vi "set_Al_PID_00.vi"(0 "target flow (sccm)":dbl=76.0 format="%.2f", 1 "Run":bool, 2 "Bubbler In":bool, 3 "Active":bool=TRUE) -> ()   [LabVIEW 2011]
uses:
  <vilib>/Analysis/NI_AALPro.lvlib
panel:
  out "prev dR":dbl
  out "dR":dbl
  out "Polynomial Coefficients":dbl[](array[numeric])=[-1.4185856873488687, 0.3207828308209371, 0.13144453708617976]
  out "Best Polynomial Fit":dbl[](array[numeric])=[-1.4185856873488687, -1.6139263817489564, -1.4535753275096295, -0.934721257482187, -0.06084472416107456, 1.168009538292087, 2.7539547788012695, 4.6979090060566655, 6.9965349595828625, 9.65378216839643, 12.656869913925354, 16.032582856357365, 19.766321537116767, 23.839791139200322, 28.29201256813708, 33.090057519195085, 38.231169600301214, 43.741895001434145, 49.604230522561835, 55.817258155180305, 63.621549699110574, 70.69684374251437, 78.07805746158404, 85.78401348130417, 93.89514333055536, 102.37353612475415, 111.1585051750553, 120.33168859799997, 129.86351160527155, 139.71949074374146, 149.9584374415381, 160.56464392932688, 171.50086747103902, 182.82343196442633, 194.50463604214053, 206.47125485701025, 218.94296295023602, 231.70008578092185, 244.74755627283324, 258.3136303817438]
  out "tFit_array":dbl[](array[numeric])=[-2.0, 0.0]
  out "RFit_array":dbl[](array[numeric])=[73.96843433835814, 74.61000000000001]
  out "error array":dbl[](array[numeric])=[-1.3899999999999864, -1.7800000000000011, -1.3500000000000085, -0.6200000000000045, 0.5699999999999932, 1.6099999999999994, 1.1999999999999886, 0.3199999999999932, -0.13000000000000966, -1.3700000000000045, -1.9499999999999886, -1.7399999999999949, -1.1200000000000045, -0.11999999999999034, 1.759999999999991, 2.3500000000000085, 2.1700000000000017, 1.4099999999999966, 0.4299999999999926, -0.6500000000000057, 54.959999999999994, 55.099999999999994, 55.66000000000001, 56.55000000000001, 57.02000000000001, 58.03, 58.129999999999995, 57.11999999999999, 56.599999999999994, 55.47, 54.80000000000001, 54.84, 55.129999999999995, 55.58, 57.16000000000001, 58.11, 58.09, 57.510000000000005, 56.74000000000001, 55.709999999999994]
  out "dt array":dbl[](array[numeric])=[0.0, -1.1669999999867287, -2.3260000000009313, -3.4940000000060536, -4.657999999995809, -5.820999999996275, -6.98499999998603, -8.14999999999418, -9.314000000013039, -10.478999999992084, -11.64000000001397, -12.807000000000698, -13.973999999987427, -15.135999999998603, -16.304000000003725, -17.469000000011874, -18.630999999993946, -19.796000000002095, -20.95999999999185, -22.122999999992317, -23.497999999992317, -24.67499999998836, -25.84299999999348, -27.005999999993946, -28.176000000006752, -29.347000000008848, -30.510999999998603, -31.679000000003725, -32.84700000000885, -34.0109999999986, -35.178000000014435, -36.345999999990454, -37.5109999999986, -38.679000000003725, -39.84700000000885, -41.00800000000163, -42.18299999998999, -43.35099999999511, -44.513000000006286, -45.68900000001304]
  out "Rtarget array":dbl[](array[numeric])=[76.0, 76.0, 76.0, 76.0, 76.0, 76.0, 76.0, 76.0, 76.0, 76.0, 76.0, 76.0, 76.0, 76.0, 76.0, 76.0, 76.0, 76.0, 76.0, 76.0, 20.0, 20.0, 20.0, 20.0, 20.0, 20.0, 20.0, 20.0, 20.0, 20.0, 20.0, 20.0, 20.0, 20.0, 20.0, 20.0, 20.0, 20.0, 20.0, 20.0]
  out "t array":dbl[](array[numeric])=[161845.394, 161844.227, 161843.068, 161841.9, 161840.736, 161839.573, 161838.409, 161837.244, 161836.08, 161834.915, 161833.754, 161832.587, 161831.42, 161830.258, 161829.09, 161827.925, 161826.763, 161825.598, 161824.434, 161823.271, 161821.896, 161820.719, 161819.551, 161818.388, 161817.218, 161816.047, 161814.883, 161813.715, 161812.547, 161811.383, 161810.216, 161809.048, 161807.883, 161806.715, 161805.547, 161804.386, 161803.211, 161802.043, 161800.881, 161799.705]
  out "R array":dbl[](array[numeric])=[74.61000000000001, 74.22, 74.64999999999999, 75.38, 76.57, 77.61, 77.19999999999999, 76.32, 75.86999999999999, 74.63, 74.05000000000001, 74.26, 74.88, 75.88000000000001, 77.75999999999999, 78.35000000000001, 78.17, 77.41, 76.42999999999999, 75.35, 74.96, 75.1, 75.66000000000001, 76.55000000000001, 77.02000000000001, 78.03, 78.13, 77.11999999999999, 76.6, 75.47, 74.80000000000001, 74.84, 75.13, 75.58, 77.16000000000001, 78.11, 78.09, 77.51, 76.74000000000001, 75.71]
  out "tuning":bool
  in  "Tune":bool
  in  "stop":bool
  in  "Ks":dbl
  out "dt(s)":dbl=1.1669999999867287
  out "windup error":dbl
  out "tPrev":dbl=161845.394
  out "target value":dbl=8.607079070006002
  out "error":dbl=-1.3899999999999864
  out "tStart(s)":dbl=161845.394
  out "weight array":dbl[](array[numeric])=[1.0, 0.3112994401423479, 0.09768570948263659, 0.03037911236430853, 0.009485414272106564, 0.0029646390229553033, 0.0009256632966347818, 0.00028873535962988374, 9.01532101455707e-05, 2.8120829299984297e-05, 8.806680295207305e-06, 2.741514645410681e-06, 8.534319742583924e-07, 2.6700458671159456e-07, 8.303530152421186e-08, 2.5900592293904588e-08, 8.103255033572197e-09, 2.5275888811806865e-09, 7.892010589399871e-10, 2.4666252724157755e-10, 6.236605368793774e-11, 1.9221339918994332e-11, 5.977611753902341e-12, 1.8682854076081917e-12, 5.79854027362869e-13, 1.7978764328562998e-13, 5.613594818436806e-14, 1.74576228867237e-14, 5.429116398891195e-15, 1.6951587510987664e-15, 5.277019701540894e-16, 1.6410913665416056e-16, 5.1189358768628024e-17, 1.5919291471855112e-17, 4.95071333304516e-18, 1.5504290109481995e-18, 4.788019052453027e-19, 1.4890178877471836e-19, 4.6585389077974155e-20, 1.437207306183795e-20]
  in  "# of points to watch":i32=60
  in  "tSmooth(s)":dbl=1.0
  out "first":bool
  out "XY Graph":cluster{"Value":dbl[], "Value":dbl[]}[](graph)=[{"Value"=[0.0, -1.1669999999867287, -2.3260000000009313, -3.4940000000060536, -4.657999999995809, -5.820999999996275, -6.98499999998603, -8.14999999999418, -9.314000000013039, -10.478999999992084, -11.64000000001397, -12.807000000000698, -13.973999999987427, -15.135999999998603, -16.304000000003725, -17.469000000011874, -18.630999999993946, -19.796000000002095, -20.95999999999185, -22.122999999992317, -23.497999999992317, -24.67499999998836, -25.84299999999348, -27.005999999993946, -28.176000000006752, -29.347000000008848, -30.510999999998603, -31.679000000003725, -32.84700000000885, -34.0109999999986, -35.178000000014435, -36.345999999990454, -37.5109999999986, -38.679000000003725, -39.84700000000885, -41.00800000000163, -42.18299999998999, -43.35099999999511, -44.513000000006286, -45.68900000001304], "Value"=[74.61000000000001, 74.22, 74.64999999999999, 75.38, 76.57, 77.61, 77.19999999999999, 76.32, 75.86999999999999, 74.63, 74.05000000000001, 74.26, 74.88, 75.88000000000001, 77.75999999999999, 78.35000000000001, 78.17, 77.41, 76.42999999999999, 75.35, 74.96, 75.1, 75.66000000000001, 76.55000000000001, 77.02000000000001, 78.03, 78.13, 77.11999999999999, 76.6, 75.47, 74.80000000000001, 74.84, 75.13, 75.58, 77.16000000000001, 78.11, 78.09, 77.51, 76.74000000000001, 75.71]}, {"Value"=[-2.0, 0.0], "Value"=[73.96843433835814, 74.61000000000001]}, {"Value"=[0.0, -1.1669999999867287, -2.3260000000009313, -3.4940000000060536, -4.657999999995809, -5.820999999996275, -6.98499999998603, -8.14999999999418, -9.314000000013039, -10.478999999992084, -11.64000000001397, -12.807000000000698, -13.973999999987427, -15.135999999998603, -16.304000000003725, -17.469000000011874, -18.630999999993946, -19.796000000002095, -20.95999999999185, -22.122999999992317, -23.497999999992317, -24.67499999998836, -25.84299999999348, -27.005999999993946, -28.176000000006752, -29.347000000008848, -30.510999999998603, -31.679000000003725, -32.84700000000885, -34.0109999999986, -35.178000000014435, -36.345999999990454, -37.5109999999986, -38.679000000003725, -39.84700000000885, -41.00800000000163, -42.18299999998999, -43.35099999999511, -44.513000000006286, -45.68900000001304], "Value"=[76.0, 76.0, 76.0, 76.0, 76.0, 76.0, 76.0, 76.0, 76.0, 76.0, 76.0, 76.0, 76.0, 76.0, 76.0, 76.0, 76.0, 76.0, 76.0, 76.0, 20.0, 20.0, 20.0, 20.0, 20.0, 20.0, 20.0, 20.0, 20.0, 20.0, 20.0, 20.0, 20.0, 20.0, 20.0, 20.0, 20.0, 20.0, 20.0, 20.0]}]
  out "current value":dbl=8.607079070006002
  in  "Period (s)":dbl=0.5
  out "dValue":dbl=2.1714937580001004
  out "derivative":dbl=0.3207828308209371
  out "integral":dbl=21701.037580001004
  in  "Kd":dbl
  in  "Ki":dbl=0.0001
  in  "Kp":dbl=0.001
  out "actual flow (sccm)":dbl=74.61000000000001 format="%.2f"
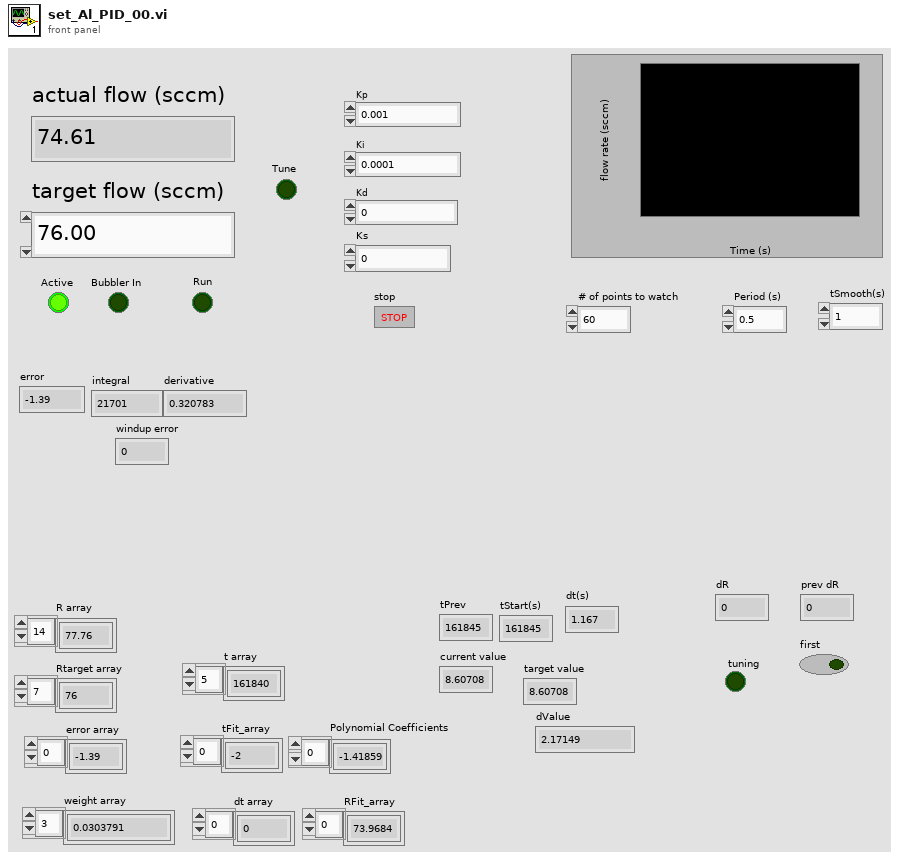
[diagram p1: front panel]
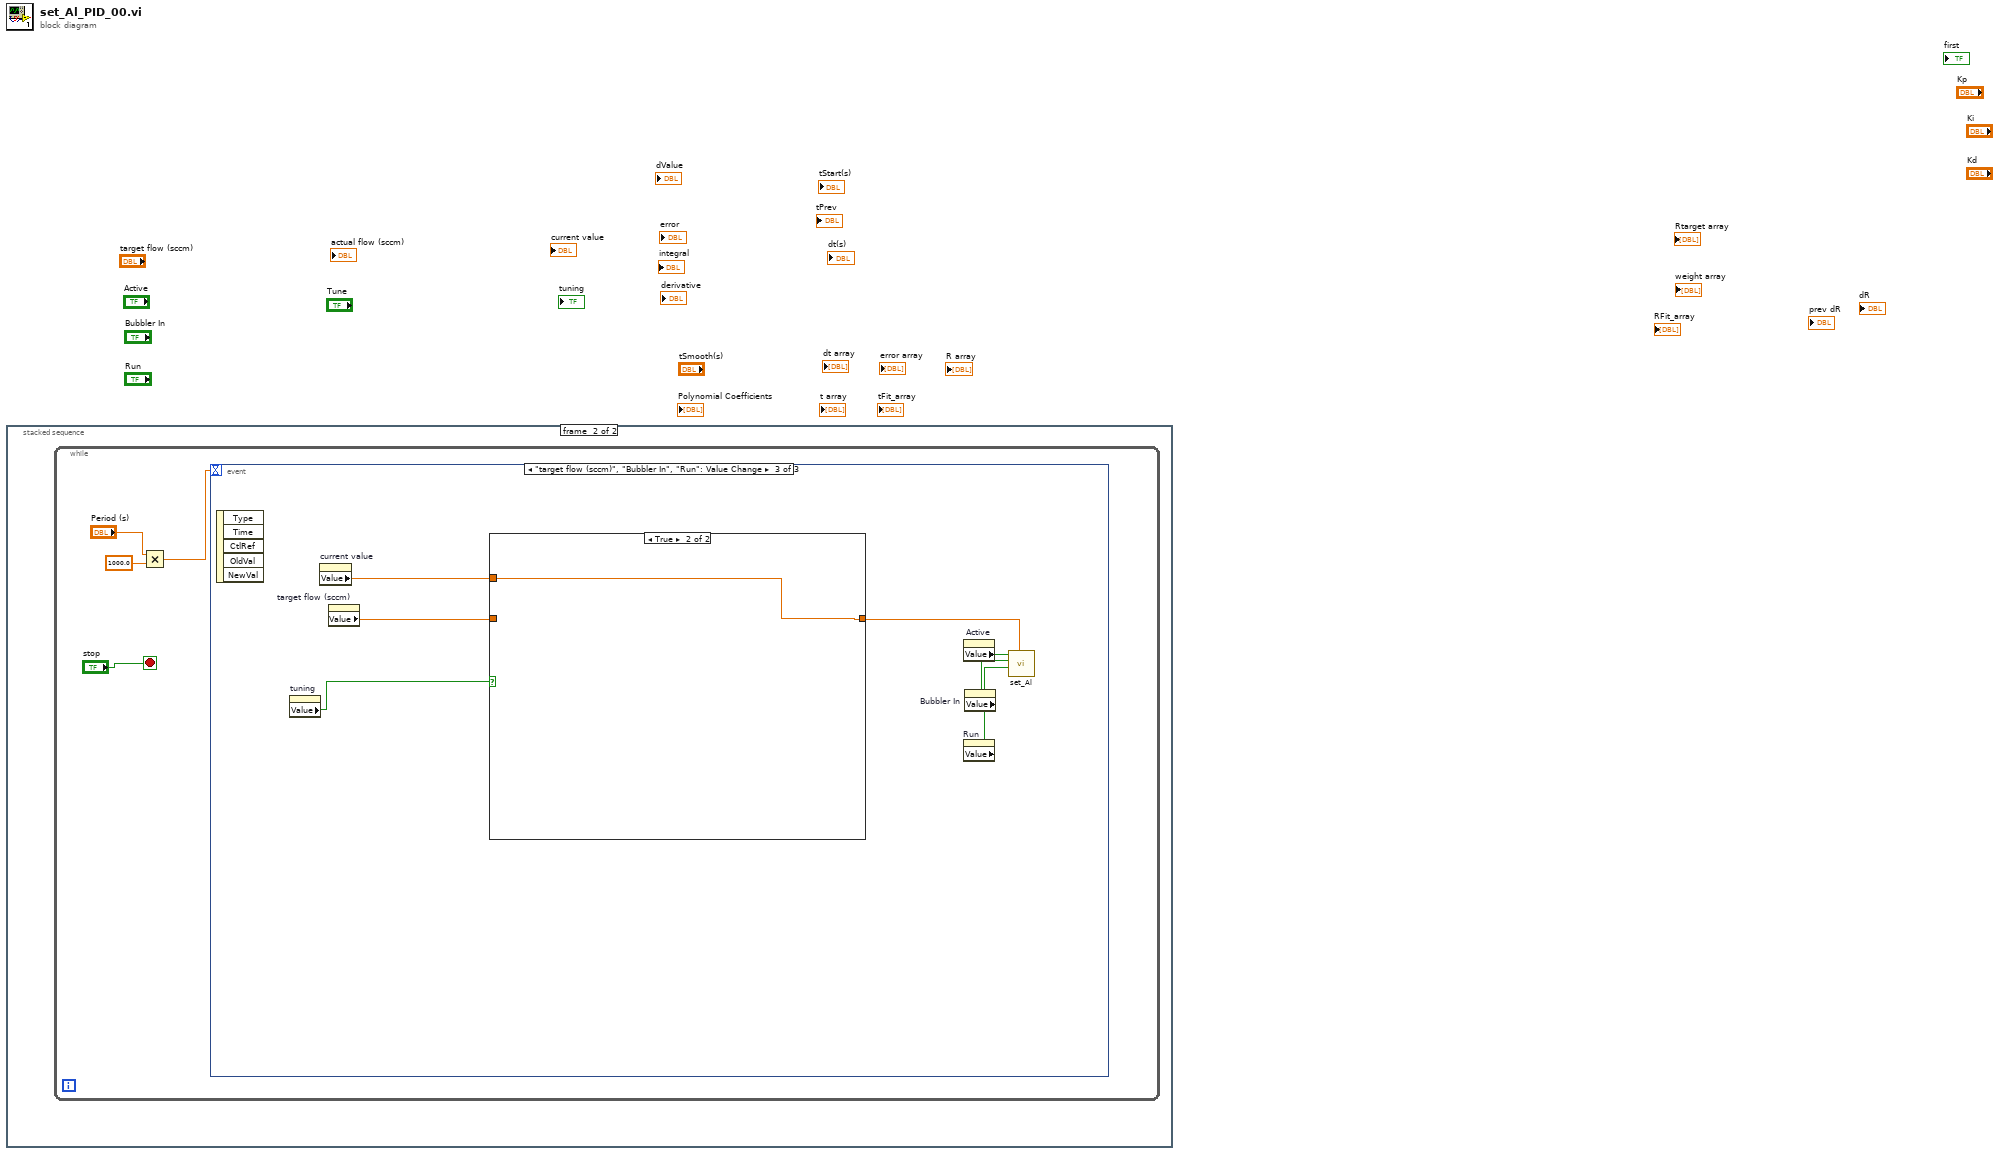
[diagram p0: block diagram]
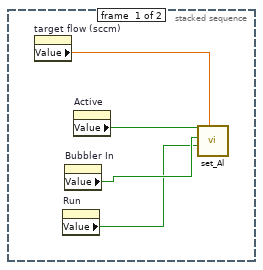
[diagram p2: hidden frame]
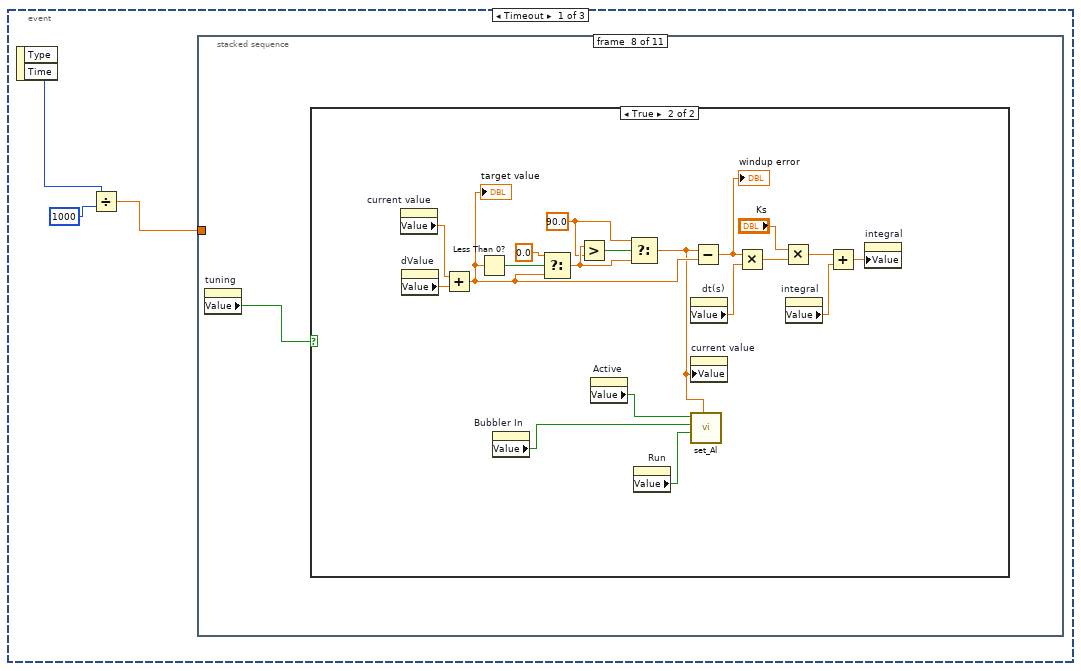
[diagram p3: hidden frame]
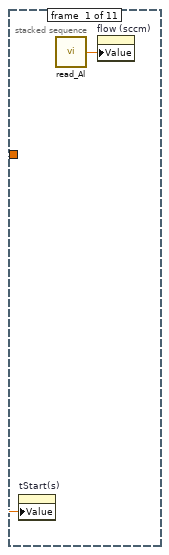
[diagram p4: hidden frame]
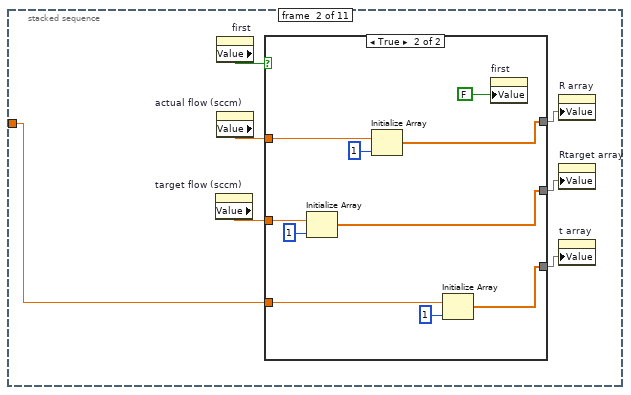
[diagram p5: hidden frame]
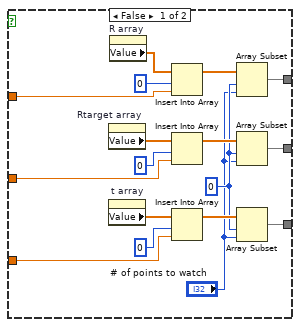
[diagram p6: hidden frame]
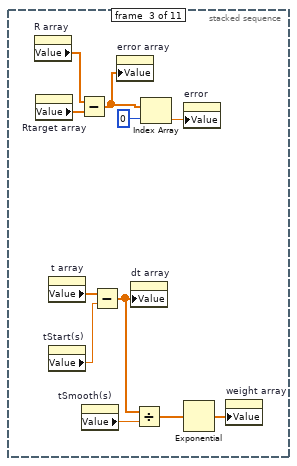
[diagram p7: hidden frame]
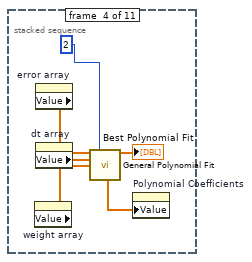
[diagram p8: hidden frame]
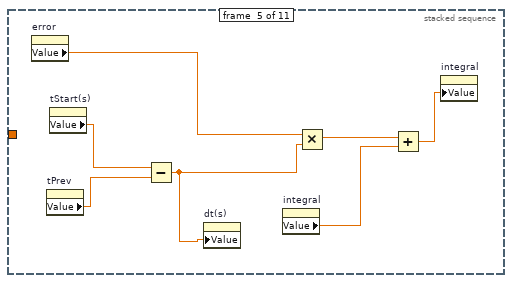
[diagram p9: hidden frame]
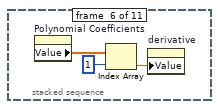
[diagram p10: hidden frame]
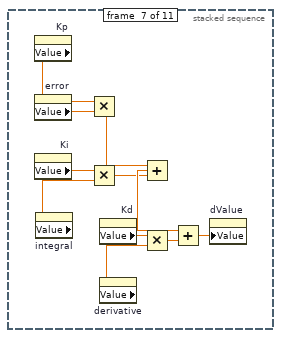
[diagram p11: hidden frame]
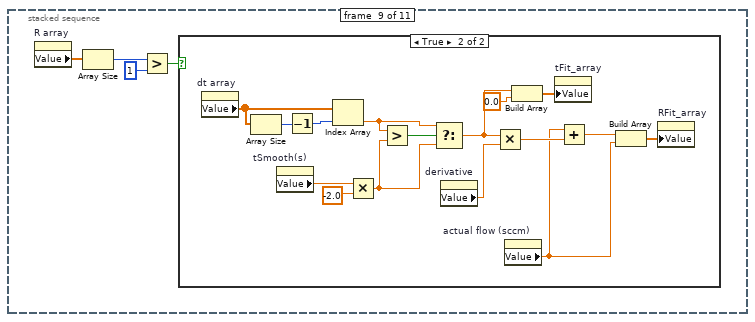
[diagram p13: hidden frame]
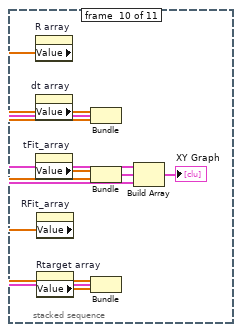
[diagram p15: hidden frame]
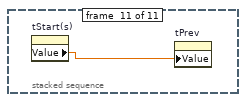
[diagram p16: hidden frame]
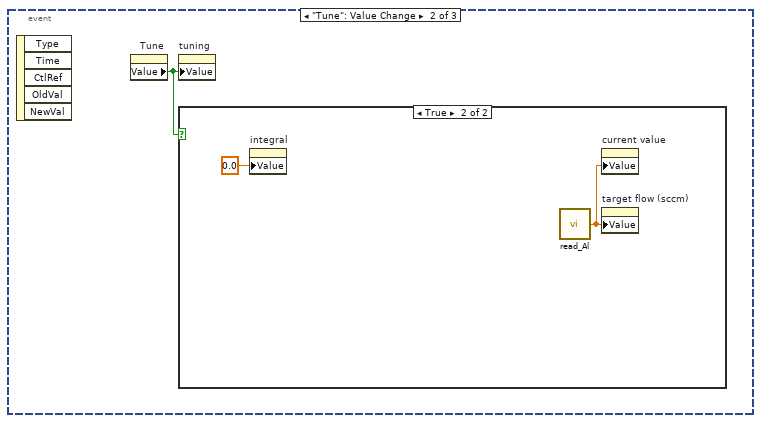
[diagram p17: hidden frame]
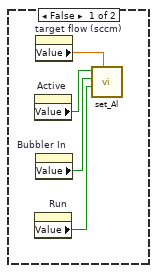
[diagram p18: hidden frame]
diagram:
  n1 = stacked-sequence {
    frame #0 {
      n2 = property on="target flow (sccm)" class="DigNum (strict)"() -> ("Value"=w2:dbl)  [unwired: 2 in, 2 out]
      n3 = property on="Run" class="Bool (strict)"() -> ("Value"=w1:bool)  [unwired: 2 in, 2 out]
      n4 = property on="Bubbler In" class="Bool (strict)"() -> ("Value"=w3:bool)  [unwired: 2 in, 2 out]
      n5 = property on="Active" class="Bool (strict)"() -> ("Value"=w4:bool)  [unwired: 2 in, 2 out]
      n6 = call "set_Al.vi"("ALMFC1"=w2, "Run"=w1, "Bubbler In"=w3, "Active"=w4) -> ()  [unwired: 6 in]
    }
    frame #1 {
      n7 = while {
        stop <- "stop" stop-if-true
        n8 = Multiply(x="Period (s)", y=1000.0) -> (x*y=w6:dbl)
        n9 = event shown="[2] \"target flow (sccm)\", \"Bubbler In\", \"Run\": Value Change" {
          selector: _ -> [_ _ _]
          dyn-events: _ -> [_ _ _]
          timeout: w6 -> [_ _ _]
          event Timeout {
            n10 = event-data() -> ("Time"=w11:u32)  [unwired: 1 in, 1 out]
            n11 = Divide(x=w11, y=u32 1000) -> (x/y=w9:dbl)
            n12 = stacked-sequence {
              tunnel: w9 -> [w13 w20 _ _ _ _ _ _ _ _ _]
              frame #0 {
                n13 = property on="tStart(s)" class="DigNum (strict)"("Value"=w13) -> ()  [unwired: 2 in, 2 out]
                n14 = call "read_Al.vi"() -> ("ALMFC1"=w12:dbl)  [unwired: 4 out]
                n15 = property on="flow (sccm)" class="DigNum (strict)"("Value"=w12) -> ()  [unwired: 2 in, 2 out]
              }
              frame #1 {
                n16 = property on="target flow (sccm)" class="DigNum (strict)"() -> ("Value"=w15:dbl)  [unwired: 2 in, 2 out]
                n17 = property on="first" class="Bool (strict)"() -> ("Value"=w19:bool)  [unwired: 2 in, 2 out]
                n18 = property on="actual flow (sccm)" class="DigNum (strict)"() -> ("Value"=w18:dbl)  [unwired: 2 in, 2 out]
                n19 = case shown="True" w19 {
                  tunnel: w18 -> [w36 w46]
                  tunnel: [w27 w44] -> w17
                  tunnel: w20 -> [w33 w42]
                  tunnel: [w25 w41] -> w16
                  tunnel: w15 -> [w29 w39]
                  tunnel: [w23 w38] -> w14
                  frame False {
                    w22 = 0 ("index")
                    n20 = property on="Rtarget array" class="Arr (strict)"() -> ("Value"=w30:dbl[])  [unwired: 2 in, 2 out]
                    n21 = property on="t array" class="Arr (strict)"() -> ("Value"=w32:dbl[])  [unwired: 2 in, 2 out]
                    n22 = property on="R array" class="Arr (strict)"() -> ("Value"=w35:dbl[])  [unwired: 2 in, 2 out]
                    n23 = Insert Into Array(array=w35, index=0, new element=w36) -> (w28:dbl[])
                    n24 = Insert Into Array(array=w30, index=0, new element=w29) -> (w24:dbl[])
                    n25 = Insert Into Array(array=w32, index=0, new element=w33) -> (w26:dbl[])
                    n26 = Array Subset(array=w28, index=w22, length="# of points to watch") -> (w27:dbl[])
                    n27 = Array Subset(array=w24, index=w22, length="# of points to watch") -> (w23:dbl[])
                    n28 = Array Subset(array=w26, index=w22, length="# of points to watch") -> (w25:dbl[])
                  }
                  frame True {
                    n29 = Initialize Array(w39, 1 ("dimension size")) -> (w38:dbl[])
                    n30 = Initialize Array(w46, 1 ("dimension size")) -> (w44:dbl[])
                    n31 = Initialize Array(w42, 1 ("dimension size")) -> (w41:dbl[])
                    n32 = property on="first" class="Bool (strict)"("Value"=FALSE ("first")) -> ()  [unwired: 2 in, 2 out]
                  }
                }
                n33 = property on="R array" class="Arr (strict)"("Value"=w17) -> ()  [unwired: 2 in, 2 out]
                n34 = property on="Rtarget array" class="Arr (strict)"("Value"=w14) -> ()  [unwired: 2 in, 2 out]
                n35 = property on="t array" class="Arr (strict)"("Value"=w16) -> ()  [unwired: 2 in, 2 out]
              }
              frame #2 {
                n36 = property on="R array" class="Arr (strict)"() -> ("Value"=w52:dbl[])  [unwired: 2 in, 2 out]
                n37 = property on="Rtarget array" class="Arr (strict)"() -> ("Value"=w51:dbl[])  [unwired: 2 in, 2 out]
                n38 = property on="t array" class="Arr (strict)"() -> ("Value"=w58:dbl[])  [unwired: 2 in, 2 out]
                n39 = property on="tStart(s)" class="DigNum (strict)"() -> ("Value"=w57:dbl)  [unwired: 2 in, 2 out]
                n40 = Subtract(x=w52, y=w51) -> (x-y=w50:dbl[])
                n41 = property on="tSmooth(s)" class="DigNum (strict)"() -> ("Value"=w56:dbl)  [unwired: 2 in, 2 out]
                n42 = Subtract(x=w58, y=w57) -> (x-y=w54:dbl[])
                n43 = property on="error array" class="Arr (strict)"("Value"=w50) -> ()  [unwired: 2 in, 2 out]
                n44 = property on="dt array" class="Arr (strict)"("Value"=w54) -> ()  [unwired: 2 in, 2 out]
                n45 = Divide(x=w54, y=w56) -> (x/y=w55:dbl[])
                n46 = Index Array(array=w50, index=0) -> (element=w48:dbl)
                n47 = property on="error" class="DigNum (strict)"("Value"=w48) -> ()  [unwired: 2 in, 2 out]
                n48 = Exponential(1:w55) -> (0:w53:dbl[])
                n49 = property on="weight array" class="Arr (strict)"("Value"=w53) -> ()  [unwired: 2 in, 2 out]
              }
              frame #3 {
                n50 = property on="weight array" class="Arr (strict)"() -> ("Value"=w62:dbl[])  [unwired: 2 in, 2 out]
                n51 = property on="error array" class="Arr (strict)"() -> ("Value"=w64:dbl[])  [unwired: 2 in, 2 out]
                n52 = property on="dt array" class="Arr (strict)"() -> ("Value"=w63:dbl[])  [unwired: 2 in, 2 out]
                n53 = call <vilib>:"General Polynomial Fit.vi"("Y"=w64, "polynomial order"=2, "X"=w63, "Weight"=w62) -> ("Best Polynomial Fit"=→"Best Polynomial Fit":dbl[], "Polynomial Coefficients"=w59:dbl[])  [unwired: 8 in, 2 out]
                n54 = property on="Polynomial Coefficients" class="Arr (strict)"("Value"=w59) -> ()  [unwired: 2 in, 2 out]
              }
              frame #4 {
                n55 = property on="error" class="DigNum (strict)"() -> ("Value"=w67:dbl)  [unwired: 2 in, 2 out]
                n56 = property on="tPrev" class="DigNum (strict)"() -> ("Value"=w66:dbl)  [unwired: 2 in, 2 out]
                n57 = property on="tStart(s)" class="DigNum (strict)"() -> ("Value"=w65:dbl)  [unwired: 2 in, 2 out]
                n58 = Subtract(x=w65, y=w66) -> (x-y=w71:dbl)
                n59 = property on="dt(s)" class="DigNum (strict)"("Value"=w71) -> ()  [unwired: 2 in, 2 out]
                n60 = property on="integral" class="DigNum (strict)"() -> ("Value"=w69:dbl)  [unwired: 2 in, 2 out]
                n61 = Multiply(x=w67, y=w71) -> (x*y=w68:dbl)
                n62 = Add(x=w68, y=w69) -> (x+y=w70:dbl)
                n63 = property on="integral" class="DigNum (strict)"("Value"=w70) -> ()  [unwired: 2 in, 2 out]
              }
              frame #5 {
                n64 = property on="Polynomial Coefficients" class="Arr (strict)"() -> ("Value"=w74:dbl[])  [unwired: 2 in, 2 out]
                n65 = Index Array(array=w74, index=1) -> (element=w72:dbl)
                n66 = property on="derivative" class="DigNum (strict)"("Value"=w72) -> ()  [unwired: 2 in, 2 out]
              }
              frame #6 {
                n67 = property on="Kp" class="DigNum (strict)"() -> ("Value"=w75:dbl)  [unwired: 2 in, 2 out]
                n68 = property on="error" class="DigNum (strict)"() -> ("Value"=w85:dbl)  [unwired: 2 in, 2 out]
                n69 = property on="Ki" class="DigNum (strict)"() -> ("Value"=w76:dbl)  [unwired: 2 in, 2 out]
                n70 = property on="integral" class="DigNum (strict)"() -> ("Value"=w77:dbl)  [unwired: 2 in, 2 out]
                n71 = Multiply(x=w75, y=w85) -> (x*y=w80:dbl)
                n72 = Multiply(x=w76, y=w77) -> (x*y=w81:dbl)
                n73 = property on="Kd" class="DigNum (strict)"() -> ("Value"=w78:dbl)  [unwired: 2 in, 2 out]
                n74 = property on="derivative" class="DigNum (strict)"() -> ("Value"=w79:dbl)  [unwired: 2 in, 2 out]
                n75 = Add(x=w80, y=w81) -> (x+y=w83:dbl)
                n76 = Multiply(x=w78, y=w79) -> (x*y=w82:dbl)
                n77 = Add(x=w83, y=w82) -> (x+y=w84:dbl)
                n78 = property on="dValue" class="DigNum (strict)"("Value"=w84) -> ()  [unwired: 2 in, 2 out]
              }
              frame #7 {
                n79 = property on="tuning" class="Bool (strict)"() -> ("Value"=w86:bool)  [unwired: 2 in, 2 out]
                n80 = case shown="True" w86 {
                  frame False {
                  }
                  frame True {
                    w99 = 90.0 ("y")
                    n81 = property on="current value" class="DigNum (strict)"() -> ("Value"=w105:dbl)  [unwired: 2 in, 2 out]
                    n82 = property on="dValue" class="DigNum (strict)"() -> ("Value"=w104:dbl)  [unwired: 2 in, 2 out]
                    n83 = Add(x=w105, y=w104) -> (x+y=w91:dbl)
                    "target value" <- w91
                    n84 = Less Than 0?(x=w91) -> (x < 0?=w103:bool)
                    n85 = property on="Bubbler In" class="Bool (strict)"() -> ("Value"=w87:bool)  [unwired: 2 in, 2 out]
                    n86 = Select(t=0.0, s=w103, f=w91) -> (s? t:f=w100:dbl)
                    n87 = Greater?(x=w100, y=w99) -> (0:w101:bool)
                    n88 = property on="Active" class="Bool (strict)"() -> ("Value"=w88:bool)  [unwired: 2 in, 2 out]
                    n89 = Select(t=w99, s=w101, f=w100) -> (s? t:f=w90:dbl)
                    n90 = property on="Run" class="Bool (strict)"() -> ("Value"=w89:bool)  [unwired: 2 in, 2 out]
                    n91 = property on="dt(s)" class="DigNum (strict)"() -> ("Value"=w97:dbl)  [unwired: 2 in, 2 out]
                    n92 = property on="current value" class="DigNum (strict)"("Value"=w90) -> ()  [unwired: 2 in, 2 out]
                    n93 = call "set_Al.vi"("ALMFC1"=w90, "Run"=w89, "Bubbler In"=w87, "Active"=w88) -> ()  [unwired: 6 in]
                    n94 = Subtract(x=w90, y=w91) -> (x-y=w98:dbl)
                    "windup error" <- w98
                    n95 = Multiply(x=w98, y=w97) -> (x*y=w96:dbl)
                    n96 = Multiply(x="Ks", y=w96) -> (x*y=w94:dbl)
                    n97 = property on="integral" class="DigNum (strict)"() -> ("Value"=w93:dbl)  [unwired: 2 in, 2 out]
                    n98 = Add(x=w94, y=w93) -> (x+y=w92:dbl)
                    n99 = property on="integral" class="DigNum (strict)"("Value"=w92) -> ()  [unwired: 2 in, 2 out]
                  }
                }
              }
              frame #8 {
                n100 = property on="R array" class="Arr (strict)"() -> ("Value"=w106:dbl[])  [unwired: 2 in, 2 out]
                n101 = Array Size(array=w106) -> (size(s)=w107:i32)
                n102 = Greater?(x=w107, y=1) -> (0:w109:bool)
                n103 = case shown="True" w109 {
                  frame False {
                  }
                  frame True {
                    n104 = property on="dt array" class="Arr (strict)"() -> ("Value"=w117:dbl[])  [unwired: 2 in, 2 out]
                    n105 = Array Size(array=w117) -> (size(s)=w125:i32)
                    n106 = property on="tSmooth(s)" class="DigNum (strict)"() -> ("Value"=w119:dbl)  [unwired: 2 in, 2 out]
                    n107 = Decrement(x=w125) -> (x-1=w124:i32)
                    n108 = Index Array(array=w117, index=w124) -> (element=w118:dbl)
                    n109 = Multiply(x=w119, y=-2.0) -> (x*y=w110:dbl)
                    n110 = Greater?(x=w118, y=w110) -> (0:w121:bool)
                    n111 = Select(t=w118, s=w121, f=w110) -> (s? t:f=w114:dbl)
                    n112 = property on="derivative" class="DigNum (strict)"() -> ("Value"=w123:dbl)  [unwired: 2 in, 2 out]
                    n113 = Multiply(x=w114, y=w123) -> (x*y=w122:dbl)
                    n114 = property on="actual flow (sccm)" class="DigNum (strict)"() -> ("Value"=w116:dbl)  [unwired: 2 in, 2 out]
                    n115 = Build Array(w114, 0.0 ("element")) -> (w112:dbl[])
                    n116 = property on="tFit_array" class="Arr (strict)"("Value"=w112) -> ()  [unwired: 2 in, 2 out]
                    n117 = Add(x=w116, y=w122) -> (x+y=w115:dbl)
                    n118 = Build Array(w115, w116) -> (w111:dbl[])
                    n119 = property on="RFit_array" class="Arr (strict)"("Value"=w111) -> ()  [unwired: 2 in, 2 out]
                  }
                }
              }
              frame #9 {
                n120 = property on="R array" class="Arr (strict)"() -> ("Value"=w134:dbl[])  [unwired: 2 in, 2 out]
                n121 = property on="dt array" class="Arr (strict)"() -> ("Value"=w126:dbl[])  [unwired: 2 in, 2 out]
                n122 = property on="tFit_array" class="Arr (strict)"() -> ("Value"=w133:dbl[])  [unwired: 2 in, 2 out]
                n123 = property on="RFit_array" class="Arr (strict)"() -> ("Value"=w132:dbl[])  [unwired: 2 in, 2 out]
                n124 = property on="Rtarget array" class="Arr (strict)"() -> ("Value"=w128:dbl[])  [unwired: 2 in, 2 out]
                n125 = Bundle("Value"=w126, "Value"=w134) -> (w131:cluster{"Value":dbl[], "Value":dbl[]})  [unwired: 1 in]
                n126 = Bundle("Value"=w133, "Value"=w132) -> (w130:cluster{"Value":dbl[], "Value":dbl[]})  [unwired: 1 in]
                n127 = Bundle("Value"=w126, "Value"=w128) -> (w127:cluster{"Value":dbl[], "Value":dbl[]})  [unwired: 1 in]
                n128 = Build Array(w131, w130, w127) -> (→"XY Graph":cluster{"Value":dbl[], "Value":dbl[]}[])
              }
              frame #10 {
                n129 = property on="tStart(s)" class="DigNum (strict)"() -> ("Value"=w135:dbl)  [unwired: 2 in, 2 out]
                n130 = property on="tPrev" class="DigNum (strict)"("Value"=w135) -> ()  [unwired: 2 in, 2 out]
              }
            }
          }
          event "Tune": Value Change {
            n131 = event-data() -> ()  [unwired: 1 in, 5 out]
            n132 = property on="Tune" class="Bool (strict)"() -> ("Value"=w136:bool)  [unwired: 2 in, 2 out]
            n133 = property on="tuning" class="Bool (strict)"("Value"=w136) -> ()  [unwired: 2 in, 2 out]
            n134 = case shown="True" w136 {
              frame False {
                n135 = property on="Active" class="Bool (strict)"() -> ("Value"=w137:bool)  [unwired: 2 in, 2 out]
                n136 = property on="Run" class="Bool (strict)"() -> ("Value"=w139:bool)  [unwired: 2 in, 2 out]
                n137 = property on="target flow (sccm)" class="DigNum (strict)"() -> ("Value"=w140:dbl)  [unwired: 2 in, 2 out]
                n138 = property on="Bubbler In" class="Bool (strict)"() -> ("Value"=w138:bool)  [unwired: 2 in, 2 out]
                n139 = call "set_Al.vi"("ALMFC1"=w140, "Run"=w139, "Bubbler In"=w138, "Active"=w137) -> ()  [unwired: 6 in]
              }
              frame True {
                n140 = property on="integral" class="DigNum (strict)"("Value"=0.0 ("integral")) -> ()  [unwired: 2 in, 2 out]
                n141 = call "read_Al.vi"() -> ("ALMFC1"=w141:dbl)  [unwired: 4 out]
                n142 = property on="current value" class="DigNum (strict)"("Value"=w141) -> ()  [unwired: 2 in, 2 out]
                n143 = property on="target flow (sccm)" class="DigNum (strict)"("Value"=w141) -> ()  [unwired: 2 in, 2 out]
              }
            }
          }
          event "target flow (sccm)", "Bubbler In", "Run": Value Change {
            n144 = event-data() -> ()  [unwired: 1 in, 5 out]
            n145 = property on="tuning" class="Bool (strict)"() -> ("Value"=w148:bool)  [unwired: 2 in, 2 out]
            n146 = property on="current value" class="DigNum (strict)"() -> ("Value"=w143:dbl)  [unwired: 2 in, 2 out]
            n147 = property on="target flow (sccm)" class="DigNum (strict)"() -> ("Value"=w149:dbl)  [unwired: 2 in, 2 out]
            n148 = case shown="True" w148 {
              tunnel: w149 -> [w150 _]
              tunnel: [w150 w151] -> w144
              tunnel: w143 -> [_ w151]
              frame False {
              }
              frame True {
              }
            }
            n149 = property on="Active" class="Bool (strict)"() -> ("Value"=w145:bool)  [unwired: 2 in, 2 out]
            n150 = property on="Run" class="Bool (strict)"() -> ("Value"=w147:bool)  [unwired: 2 in, 2 out]
            n151 = property on="Bubbler In" class="Bool (strict)"() -> ("Value"=w146:bool)  [unwired: 2 in, 2 out]
            n152 = call "set_Al.vi"("ALMFC1"=w144, "Run"=w147, "Bubbler In"=w146, "Active"=w145) -> ()  [unwired: 6 in]
          }
        }
      }
    }
  }
